vi "Thermalwave Main.vi"() -> ()   [LabVIEW 2011]
panel:
  in  "?":bool
  out "Path":path
  out "d5":string
  out "d4":string
  out "d3":string
  out "d2":string
  out "d1":string
  out "Thermalwave Measurement":dbl[](graph)
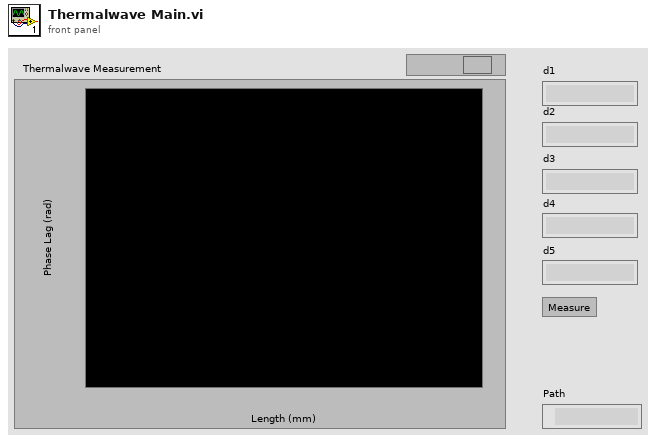
[diagram p1: front panel]
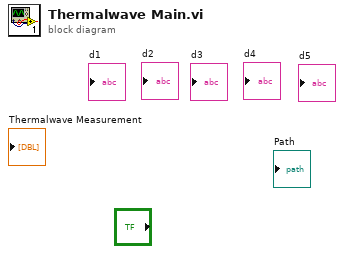
[diagram p0: block diagram]
diagram:
